vi "setUp.vi"(8 "error in (no error)":errorcluster, 11 "reference in":refnum<class "Routing and Faulting Import Unit Tests.lvclass">) -> (0 "error out":errorcluster, 3 "reference out":refnum<class "Routing and Faulting Import Unit Tests.lvclass">)   [LabVIEW 2019, in "Routing and Faulting Import Unit Tests.lvclass"]
doc: "setUp runs prior to the test method during test execution. Use this method to initialize any object data required by your tests."
uses:
  Routing and Faulting Import Unit Tests.lvclass
  <vilib>/addons/_JKI Toolkits/VI Tester/TestCase.llb/TestCase.lvclass
  <vilib>/NI/VeriStand Custom Device Testing Tools/VeriStandTestUtilities/VeriStandTestUtilities.lvlib
  <userlib>/_OpenG.lib/file/file.llb/Append Path to Root if Relative - Scalar__ogtk.vi
  NationalInstruments.VeriStand.SystemDefinitionAPI
  C:/Program Files (x86)/National Instruments/LabVIEW 2019/vi.lib/addons/_JKI Toolkits/VI Tester/TestCase.llb/TestCase.lvclass
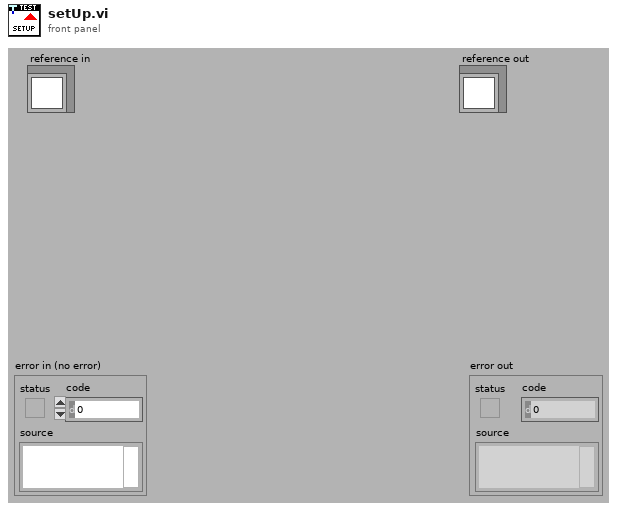
[diagram p1: front panel]
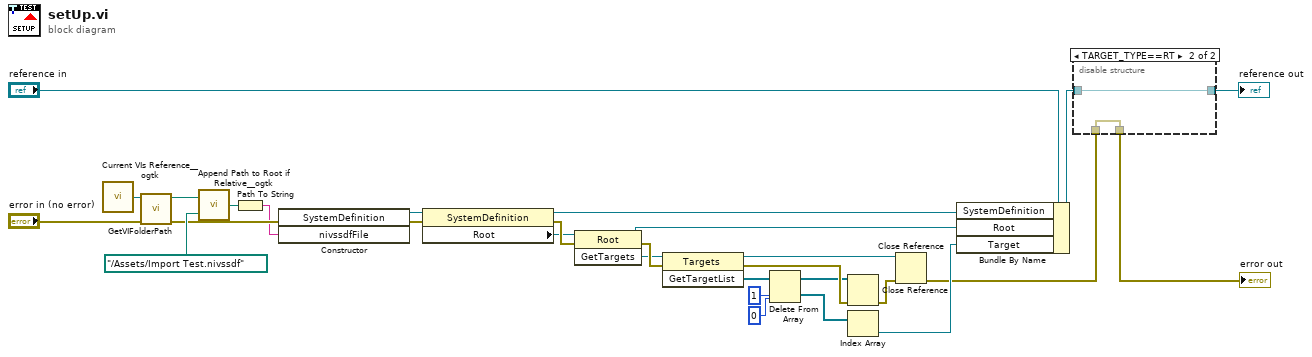
[diagram p0: block diagram]
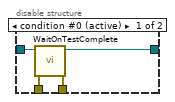
[diagram p2: hidden frame]
diagram:
  n1 = call <userlib>:"Current VIs Reference__ogtk.vi"() -> ("Current VI's reference"=w27:refnum<vi>)  [unwired: 5 in]
  n2 = call <vilib>:"GetVIFolderPath.vi"("error in (no error)"="error in (no error)", "VI Reference in"=w27) -> ("error out"=w23:errorcluster, "VI Folder Path out"=w26:path)  [unwired: 8 in]
  n3 = call-poly <userlib>:"Append Path to Root if Relative__ogtk.vi"("Absolute or Relative Path"=path "../Assets/Import Test.nivssdf", "Root Path"=w26) -> ("Absolute or Appended Path"=w24:path)
  n4 = Path To String(path=w24) -> (string=w21:string)
  n5 = constructor class="SystemDefinition"(error in=w23, "nivssdfFile"=w21) -> (reference out=w20:refnum<k24>, error out=w22:errorcluster)  [unwired: 2 in, 2 out]
  n6 = property class="SystemDefinition"(reference=w20, error in=w22) -> (reference out=w5:refnum<k24>, error out=w19:errorcluster, "Root"=w18:refnum<k24>)
  n7 = invoke class="Root" method="GetTargets"(reference=w18, error in=w19) -> (reference out=w6:refnum<k24>, error out=w17:errorcluster, "GetTargets"=w16:refnum<k24>)  [unwired: 1 in]
  n8 = invoke class="Targets" method="GetTargetList"(reference=w16, error in=w17) -> (reference out=w9:refnum<k24>, error out=w12:errorcluster, "GetTargetList"=w15:refnum<k24>[])  [unwired: 1 in]
  n9 = Delete From Array(array=w15, length=1, index=0) -> (deleted portion=w8:refnum<k24>[], array with subset deleted=w11:refnum<k24>[])
  n10 = Close Reference(reference=w11, error in (no error)=w12) -> (error out=w10:errorcluster)
  n11 = Index Array(array=w8) -> (element=w7:refnum<k24>)  [unwired: 1 in]
  n12 = Close Reference(reference=w9, error in (no error)=w10) -> (error out=w1:errorcluster)
  n13 = Bundle By Name(cluster="reference in", "SystemDefinition"=w5, "Root"=w6, "Target"=w7) -> (w3:refnum<class "Routing and Faulting Import Unit Tests.lvclass">)
  n14 = disable-structure shown="TARGET_TYPE==RT" {
    disable-tunnel: w1 -> [w33 w34]
    disable-tunnel: [w32 w34] -> w29
    disable-tunnel: [w31 w35] -> w28
    disable-tunnel: w3 -> [w30 w35]
    frame condition #0 (active) {
      n15 = call <vilib>:"WaitOnTestComplete.vi"("error in (no error)"=w33, "TestCase in"=w30) -> ("error out"=w32:errorcluster, "TestCase out"=w31:refnum<class "Routing and Faulting Import Unit Tests.lvclass">)  [unwired: 8 in]
    }
    frame condition #1 {
    }
  }
  "error out" <- w29
  "reference out" <- w28
